vi "FPGA_read.vi"() -> ()   [LabVIEW 2020]
uses:
  <vilib>/rvi/eio/common/nirviEmuTemplateMethod_errors.vi
  <vilib>/rvi/interface/RandomDataEmulation/niFpgaRandomDataHandleErrors.vi
  <vilib>/eio/EIONode/EIONode.xnode
  <vilib>/rvi/DataTransferAndStorage/Container/XNode/niFpgaContainer.xnode
  <vilib>/rvi/interface/RandomDataEmulation/nirviRandomDataFpgaReadWriteTemplate.vi
panel:
  in  "Loop number":i32
  out "Element":fxp<+/-,24,7>
  out "Actual loop rate":u32
  in  "Rate (uSec)":u32 caption="Count(uSec)"
  out "Timed Out?":bool
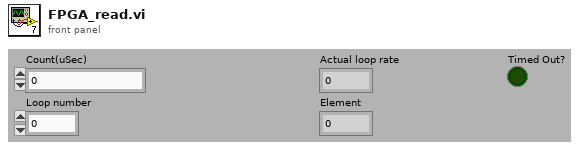
[diagram p1: front panel]
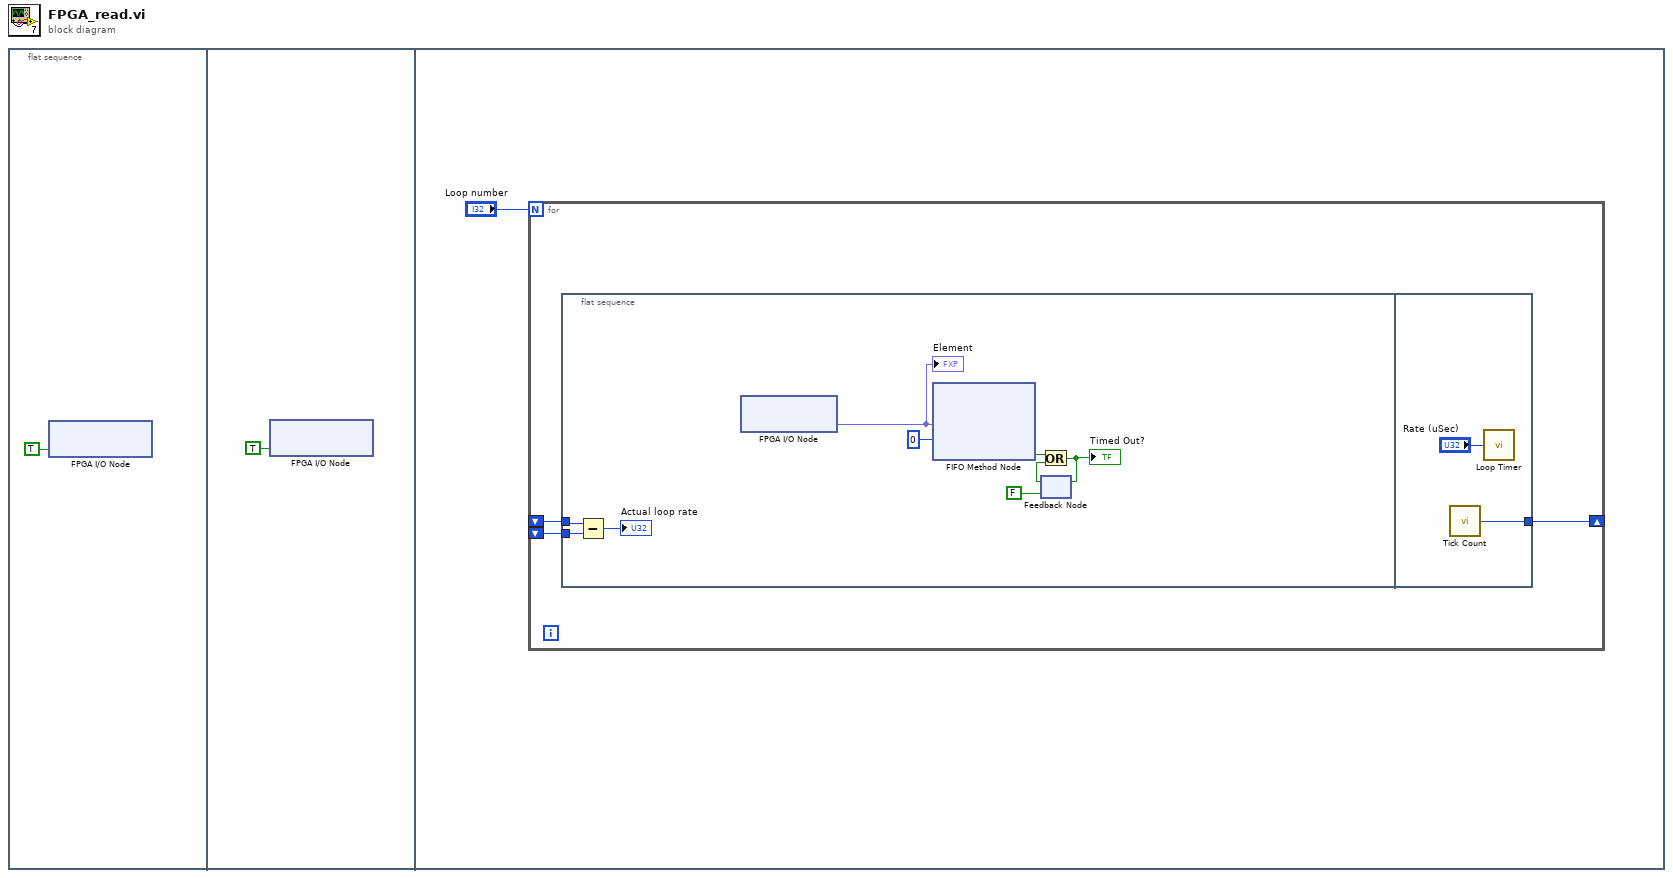
[diagram p0: block diagram]
diagram:
  n1 = flat-sequence {
    frame #0 {
      n2 = xnode "FPGA I/O Node"("Mod1/Stop"=TRUE) -> ()  [unwired: 1 in, 1 out]
    }
    frame #1 {
      n3 = xnode "FPGA I/O Node"("Mod1/Start"=TRUE) -> ()  [unwired: 1 in, 1 out]
    }
    frame #2 {
      n4 = for {
        N: "Loop number" -> [_]
        shift-right: [w6] -> _
        shift-left: _ -> [w5]
        shift-left: _ -> [w4]
        n5 = flat-sequence {
          tunnel: w5 -> [w15]
          tunnel: w4 -> [w14]
          tunnel: [w16] -> w6
          frame #0 {
            n6 = Subtract(x=w15, y=w14) -> (x-y=→"Actual loop rate":u32)
            n7 = xnode "FPGA I/O Node"() -> ("Mod1/AI0"=w7:fxp<+/-,24,7>)  [unwired: 1 in, 1 out]
            "Element" <- w7
            n8 = xnode ("FIFO Method Node")("Element"=w7, "Timeout"=0) -> ("Timed Out?"=w11:bool)  [unwired: 2 in, 2 out]
            n9 = feedback #1(FALSE) -> (w10:bool)
            n10 = Or(x=w11, y=w10) -> (x .or. y?=w9:bool)
            "Timed Out?" <- w9
            n11 = feedback-in #1(w9) -> ()
          }
          frame #1 {
            n12 = call "Tick Count"() -> ("Tick Count(uSec)"=w16:u32)
            n13 = call "Loop Timer"("Count(uSec)"="Rate (uSec)") -> ()  [unwired: 1 out]
          }
        }
      }
    }
  }
